vi "VarInterface_DoScripting.vi"(0 "diagram":refnum<vi>, 1 "ScriptingRules":T5, 5 "VariableTerminals":T1, 7 "variable":T2, 9 "URL":string, 11 "error in":errorcluster, 12 "XRef":refnum<vi>) -> (15 "error out":errorcluster)   [LabVIEW 2017, in "NI_Variable.lvlib"]
doc: "Script the runtime behavior for the variable"
uses:
  <vilib>/variable/NI_Variable.lvlib
  <vilib>/variable/ScriptingRules.ctl
  <vilib>/variable/variable.ctl
  <vilib>/variable/Type Descriptor.ctl
  <vilib>/variable/Attribs.ctl
  <vilib>/variable/VariableTerminals.ctl
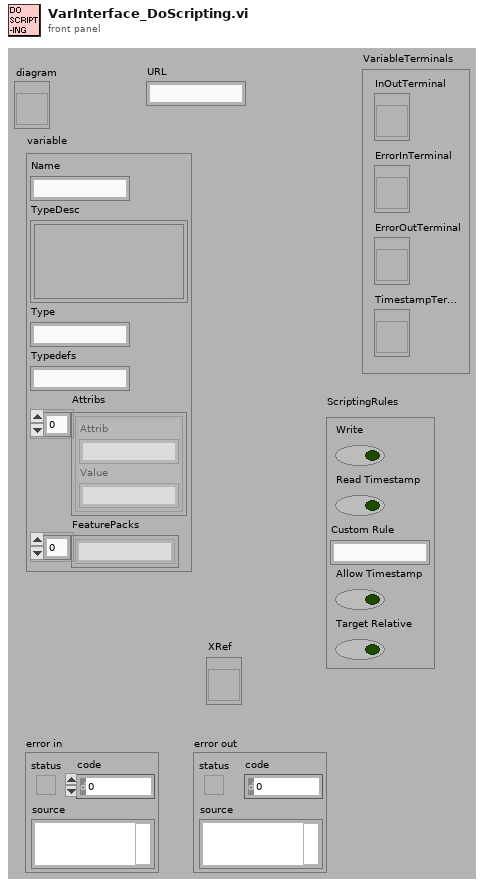
[diagram p1: front panel]
types:
  T1 = typedef "NI_Variable.lvlib/VariableTerminals.ctl" = cluster{"InOutTerminal":refnum<vi>, "ErrorInTerminal":refnum<vi>, "ErrorOutTerminal":refnum<vi>, "TimestampTerminal":refnum<vi>}
  T2 = typedef "NI_Variable.lvlib/variable.ctl" = cluster{"Name":string, "TypeDesc":T3, "Type":string, "Typedefs":string, "Attribs":T4, "FeaturePacks":string[]}
  T3 = typedef "NI_Variable.lvlib/Type Descriptor.ctl" = cluster{"Variant":variant}
  T4 = typedef "NI_Variable.lvlib/Attribs.ctl" = cluster{"Attrib":string, "Value":string}[]
  T5 = typedef "NI_Variable.lvlib/ScriptingRules.ctl" = cluster{"Write":bool, "Read Timestamp":bool, "Custom Rule":string, "Allow Timestamp":bool, "Target Relative":bool}
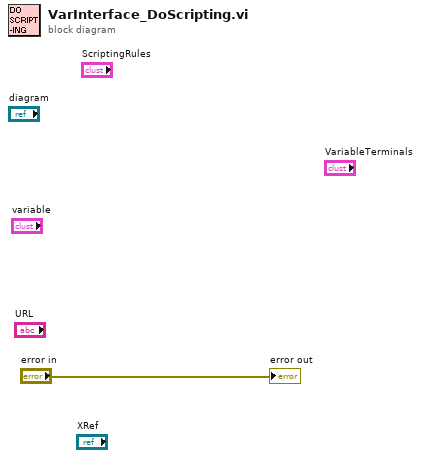
[diagram p0: block diagram]
diagram:
  "error out" <- "error in"
